vi "c Spark Safe Float.vi"(8 "error in (no error)":errorcluster, 11 "f":sgl) -> (0 "error out":errorcluster, 3 "function return":sgl)   [LabVIEW 2023, in "REVLibDriver.lvlib"]
doc: "float c_Spark_SafeFloat(float f);"
uses:
  REVLibDriver.lvlib
  REVLibDriver.dll
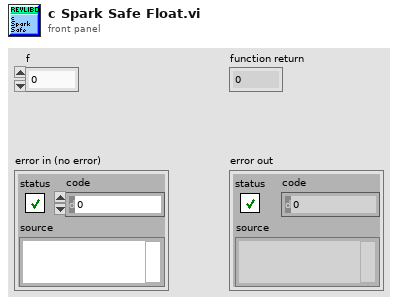
[diagram p1: front panel]
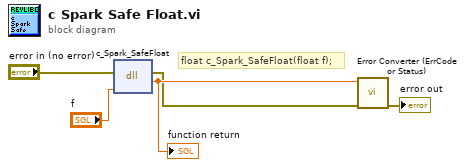
[diagram p0: block diagram]
diagram:
  # "float c_Spark_SafeFloat(float f);"
  n1 = dll-call lib="REVLibDriver.*" fn="c_Spark_SafeFloat"(error in="error in (no error)", "f"="f") -> (error out=w2:errorcluster, w5:sgl)  [unwired: 3 in, 1 out]
  "function return" <- w5
  n2 = call "Error Converter (ErrCode or Status).vi"("error in (no error)"=w2, "error code"=w5) -> ("error out"=→"error out":errorcluster)  [unwired: 9 in]
